vi "Intake Execute.vi"() -> ()   [LabVIEW 2017]
uses:
  Intake Control Type.ctl
  <vilib>/Rock Robotics/WPI/Solenoid/WPI_SolenoidValue.ctl
  <vilib>/Rock Robotics/WPI/DriverStation/WPI_DriverStationRobotMode2.ctl
  Intake Notifier.ctl
  <vilib>/Rock Robotics/WPI/ThirdParty/Phoenix-LabVIEW/Motor Controller/Controls/CTRE_Phoenix_MotorControl_ControlMode.ctl
  Intake Globals.vi
  Utility VIs/Refnum Names.vi
  Robot Global Data.vi
  Lift/Lift Globals.vi
  <vilib>/Rock Robotics/Network Tables/NT Write Boolean.vi
  <vilib>/Rock Robotics/WPI/Solenoid/WPI_SolenoidSetEnum.vi
  Intake Rotation/Intake Rotation Globals.vi
panel:
  in  "Max Out":dbl=0.65 format="%#_13g"
  in  "Arm Out Engaged":bool
  out "error out 3":errorcluster
  out "error out 2":errorcluster
  out "error out":errorcluster
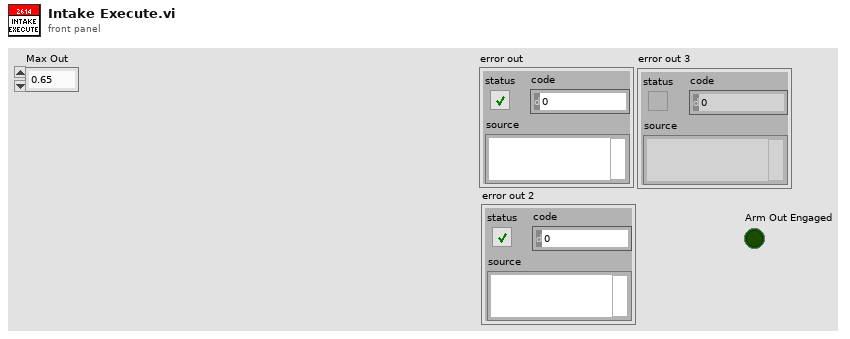
[diagram p1: front panel]
types:
  T1 = typedef "WPI_SolenoidDevRef.ctl" = cluster{"DevStatus":errorcluster, "Pneumatics Control Module":u8, "Forward Solenoid Channel":T2, "Reverse Solenoid Channel":T2}
  T2 = typedef "WPI_SolenoidChannel.ctl" = enum8{"Solenoid 0", "Solenoid 1", "Solenoid 2", "Solenoid 3", "Solenoid 4", "Solenoid 5", "Solenoid 6", "Solenoid 7", "Invalid"}
  T3 = typedef "WPI_MotorControlDeviceRef.ctl" = cluster{"DeviceStatus":errorcluster, "Type":T4, "PWM":cluster{"PWM Channel":T5, "DeadBand":T6}, "CAN":cluster{"Device Number":u8, "SetOutput VI Ref":variant, "GetOutput VI Ref":variant, "Enable VI Ref":variant, "Disable VI Ref":variant, "Data":variant}, "Invert":bool, "DIO PWM":cluster{"PWM \"Enable\" Channel":T5, "DIOChannel":T7, "PWM Rate":dbl}}
  T4 = typedef "WPI_MotorControlType.ctl" = enum16{"PWM", "CAN", "DIO PWM"}
  T5 = typedef "FPGA_DIOPWMChannel.ctl" = enum8{"PWM 0", "PWM 1", "PWM 2", "PWM 3", "PWM 4", "PWM 5", "PWM 6", "PWM 7", "PWM 8", "PWM 9", "PWM MXP 0", "PWM MXP 1", "PWM MXP 2", "PWM MXP 3", "PWM MXP 4", "PWM MXP 5", "PWM MXP 6", "PWM MXP 7", "PWM MXP 8", "PWM MXP 9", "Invalid"}
  T6 = typedef "WPI_PWMDeadband.ctl" = cluster{"Name":string, "maxPositivePwm":i32, "minPositivePwm":i32, "centerPwm":i32, "maxNegativePwm":i32, "minNegativePwm":i32, "angularRange":u16}
  T7 = typedef "FPGA_DIOChannel.ctl" = enum8{"DIO 0", "DIO 1", "DIO 2", "DIO 3", "DIO 4", "DIO 5", "DIO 6", "DIO 7", "DIO 8", "DIO 9", "DIO MXP 0", "DIO MXP 1", "DIO MXP 2", "DIO MXP 3", "DIO MXP 4", "DIO MXP 5", "DIO MXP 6", "DIO MXP 7", "DIO MXP 8", "DIO MXP 9", "DIO MXP 10", "DIO MXP 11", "DIO MXP 12", "DIO MXP 13", "DIO MXP 14", "DIO MXP 15", "SPI Port CS1", "SPI Port CS2", "SPI Port CS3", "SPI Port MISO", "SPI Port MOSI", "Invalid"}
  T8 = typedef "WPI_DriverStationRobotMode2.ctl" = enum16{"Autonomous Disabled", "Autonomous Enabled", "Teleop Disabled", "Teleop Enabled", "Disconnected", "Finish", "Test Disabled", "Test Enabled", "Emergency Stopped"}
  T9 = typedef "WPI_SolenoidValue.ctl" = enum16{"Off", "On", "Forward", "Reverse"}
  T10 = typedef "Intake Control Type.ctl" = enum16{"No Op", "In", "Out", "Test Mode", "Cube_In", "Cube_Out", "State_Change"}
  T11 = typedef "Intake Notifier.ctl" = cluster{"Intake Control Type":T10, "Step":i32, "In":bool, "Speed":dbl, "Out":bool, "Parameter 1":dbl, "Parameter 2":dbl, "Intake Notifier":refnum<notifier>, "Actuate Cube":bool, "Speed In":dbl, "Speed Out":dbl, "Load":bool, "Override":bool, "Exchange":bool, "Intake Open":bool}
  T12 = typedef "CTRE_Phoenix_MotorControl_ControlMode.ctl" = u16
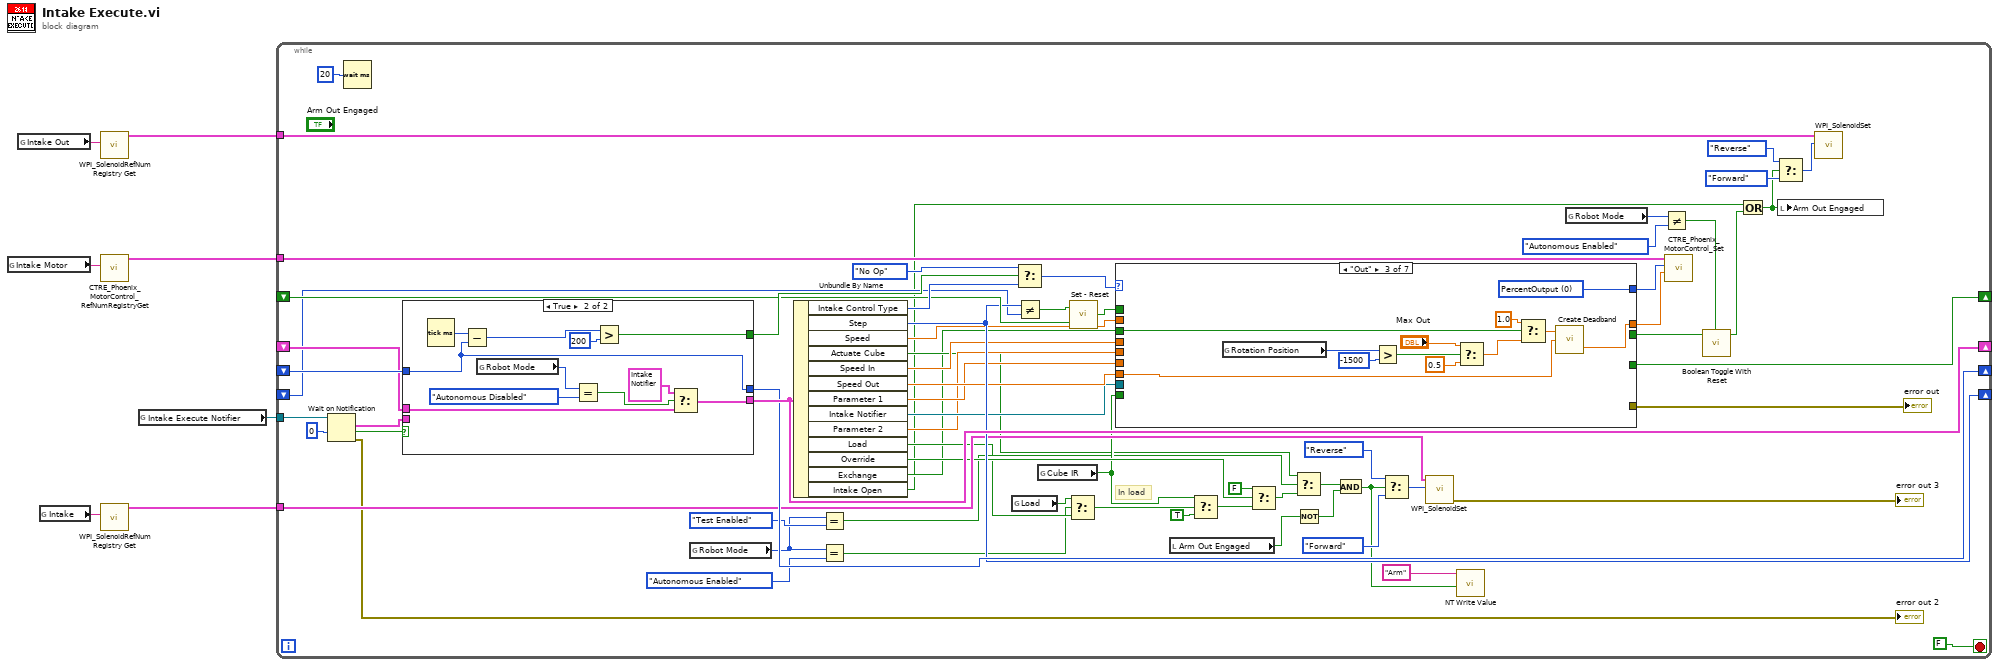
[diagram p0: block diagram]
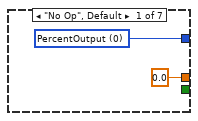
[diagram p2: hidden frame]
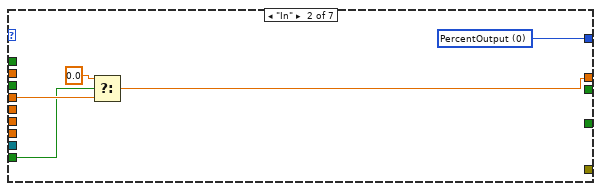
[diagram p3: hidden frame]
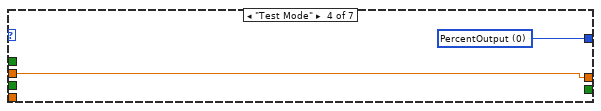
[diagram p4: hidden frame]
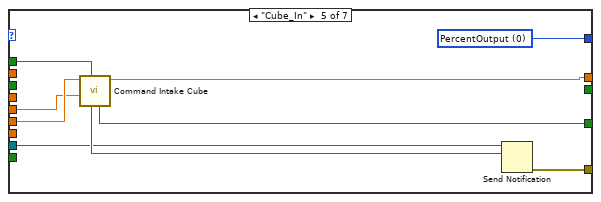
[diagram p5: hidden frame]
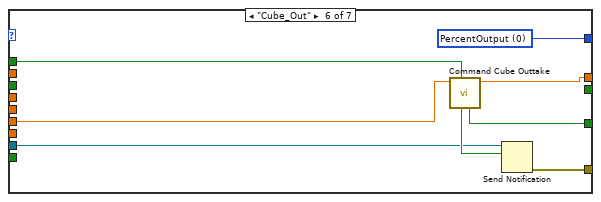
[diagram p6: hidden frame]
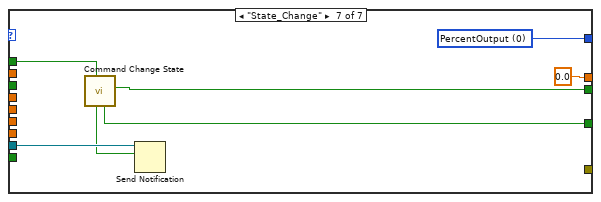
[diagram p7: hidden frame]
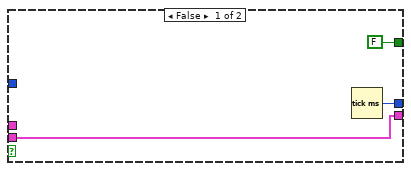
[diagram p8: hidden frame]
diagram:
  n1 = global read "Refnum Names.vi" "Intake Motor"() -> (w6:string)
  n2 = global read "Refnum Names.vi" "Intake Out"() -> (w2:string)
  n3 = global read "Refnum Names.vi" "Intake"() -> (w4:string)
  n4 = call <vilib>:"WPI_SolenoidRefNum Registry Get.vi"("refnum name"=w2) -> ("SolenoidDevRef"=w1:T1)  [unwired: 9 in, 1 out]
  n5 = call <vilib>:"CTRE_Phoenix_MotorControl_RefNumRegistryGet.vi"("refnum name"=w6) -> ("PhoenixMotorControlDevRef"=w5:T3)  [unwired: 9 in, 1 out]
  n6 = call <vilib>:"WPI_SolenoidRefNum Registry Get.vi"("refnum name"=w4) -> ("SolenoidDevRef"=w3:T1)  [unwired: 9 in, 1 out]
  n7 = global read "Intake Globals.vi" "Intake Execute Notifier"() -> (w7:refnum<notifier>)
  n8 = while {
    tunnel: w7 -> [w73]
    shift-right: [w69] -> _
    shift-left: _ -> [w63]
    shift-right: [w67] -> _
    shift-left: _ -> [w68]
    shift-right: [w59] -> _
    shift-left: _ -> [w58]
    shift-right: [w57] -> _
    shift-left: _ -> [w56]
    tunnel: w5 -> [w55]
    tunnel: w3 -> [w51]
    tunnel: w1 -> [w20]
    stop <- FALSE stop-if-true
    # "In load"
    n9 = Wait on Notification(notifier=w73, timeout in ms (-1)=0) -> (notification=w70:T11, timed out?=w71:bool, error out=→"error out 2":errorcluster)  [unwired: 2 in, 1 out]
    n10 = Wait (ms)(milliseconds to wait=u32 20) -> ()  [unwired: 1 out]
    n11 = case shown="True" w71 {
      tunnel: [w122 w129] -> w69
      tunnel: w70 -> [w122 _]
      tunnel: w68 -> [_ w131]
      tunnel: [w123 w131] -> w67
      tunnel: [FALSE w130] -> w64
      tunnel: w63 -> [_ w128]
      frame False {
        n12 = Tick Count (ms)() -> (millisecond timer value=w123:u32)
      }
      frame True {
        n13 = Tick Count (ms)() -> (millisecond timer value=w134:u32)
        n14 = Subtract(x=w134, y=w131) -> (x-y=w133:u32)
        n15 = global read "Robot Global Data.vi" "Robot Mode"() -> (w126:T8)
        n16 = Equal?(x=w126, y=WPI_DriverStationRobotMode2."Autonomous Disabled") -> (x = y?=w124:bool)
        n17 = Greater?(x=w133, y=u32 200) -> (0:w130:bool)
        n18 = Select(t=T11 {"Intake Control Type"=enum."No Op", "Step"=0, "In"=FALSE, "Speed"=0.0, "Out"=FALSE, "Parameter 1"=0.0, "Parameter 2"=0.0, "Intake Notifier"=refnum, "Actuate Cube"=FALSE, "Speed In"=0.0, "Speed Out"=0.0, "Load"=FALSE, "Override"=FALSE, "Exchange"=FALSE, "Intake Open"=FALSE} ("Intake Notifier"), s=w124, f=w128) -> (s? t:f=w129:T11)
      }
    }
    n19 = global read "Robot Global Data.vi" "Robot Mode"() -> (w24:T8)
    n20 = Unbundle By Name(w69) -> ("Intake Control Type"=w65:T10, "Step"=w57:i32, "Speed"=w52:dbl, "Actuate Cube"=w33:bool, "Speed In"=w47:dbl, "Speed Out"=w46:dbl, "Parameter 1"=w45:dbl, "Intake Notifier"=w44:refnum<notifier>, "Parameter 2"=w43:dbl, "Load"=w28:bool, "Override"=w40:bool, "Exchange"=w22:bool, "Intake Open"=w14:bool)
    n21 = Equal?(x=w24, y=WPI_DriverStationRobotMode2."Test Enabled") -> (x = y?=w35:bool)
    n22 = Equal?(x=w24, y=WPI_DriverStationRobotMode2."Autonomous Enabled") -> (x = y?=w25:bool)
    n23 = global read "Lift Globals.vi" "Load"() -> (w23:bool)
    n24 = Select(t=Intake_Control_Type."No Op", s=w64, f=w65) -> (s? t:f=w66:T10)
    n25 = Not Equal?(x=w57, y=w56) -> (x != y?=w61:bool)
    n26 = global read "Intake Globals.vi" "Cube IR"() -> (w39:bool)
    n27 = Select(t=w23, s=w25, f=w28) -> (s? t:f=w27:bool)
    n28 = call "Set - Reset.vi"("Reset"=w58, "Set"=w61) -> ("Output"=w60:bool)
    n29 = case shown="\"Out\"" w66 {
      tunnel: w60 -> [_ _ _ _ w103 w108 w115]
      tunnel: [_ _ _ _ w100 w112 w118] -> w59
      tunnel: [0.0 ("Output") w80 w92 w95 w105 w113 0.0 ("Output")] -> w54
      tunnel: [w76 w82 w94 w96 w104 w107 w120] -> w53
      tunnel: w52 -> [_ _ _ w95 _ _ _]
      tunnel: w47 -> [_ w81 _ _ _ _ _]
      tunnel: w39 -> [_ w79 _ _ _ _ _]
      tunnel: w46 -> [_ _ w93 _ _ _ _]
      tunnel: w45 -> [_ _ _ _ w102 w109 _]
      tunnel: w44 -> [_ _ _ _ w99 w110 w117]
      tunnel: w43 -> [_ _ _ _ w98 _ _]
      tunnel: [_ _ _ _ w97 w106 _] -> w42
      tunnel: w22 -> [_ _ w89 _ _ _ _]
      tunnel: [_ _ _ _ _ _ w114] -> w12
      frame "No Op", Default {
        w76 = T12 0 items=["PercentOutput"=0, "Position"=1, "Velocity"=2, "Current"=3, "Follower"=5, "MotionProfile"=6, "MotionMagic"=7, "MotionMagicArc"=8, "MotionProfileArc"=10, "Disabled"=15] ("Control Mode")
      }
      frame "In" {
        w82 = T12 0 items=["PercentOutput"=0, "Position"=1, "Velocity"=2, "Current"=3, "Follower"=5, "MotionProfile"=6, "MotionMagic"=7, "MotionMagicArc"=8, "MotionProfileArc"=10, "Disabled"=15] ("Control Mode")
        n30 = Select(t=0.0, s=w79, f=w81) -> (s? t:f=w80:dbl)
      }
      frame "Out" {
        w94 = T12 0 items=["PercentOutput"=0, "Position"=1, "Velocity"=2, "Current"=3, "Follower"=5, "MotionProfile"=6, "MotionMagic"=7, "MotionMagicArc"=8, "MotionProfileArc"=10, "Disabled"=15] ("Control Mode")
        n31 = global read "Intake Rotation Globals.vi" "Rotation Position"() -> (w86:i32)
        n32 = Greater?(x=w86, y=-1500) -> (0:w87:bool)
        n33 = Select(t="Max Out", s=w87, f=0.5) -> (s? t:f=w88:dbl)
        n34 = Select(t=1.0, s=w89, f=w88) -> (s? t:f=w91:dbl)
        n35 = call "Create Deadband.vi"("Input"=w93, "Output Upper Limit"=w91) -> ("Output"=w92:dbl)  [unwired: 2 in]
      }
      frame "Test Mode" {
        w96 = T12 0 items=["PercentOutput"=0, "Position"=1, "Velocity"=2, "Current"=3, "Follower"=5, "MotionProfile"=6, "MotionMagic"=7, "MotionMagicArc"=8, "MotionProfileArc"=10, "Disabled"=15] ("Control Mode")
      }
      frame "Cube_In" {
        w104 = T12 0 items=["PercentOutput"=0, "Position"=1, "Velocity"=2, "Current"=3, "Follower"=5, "MotionProfile"=6, "MotionMagic"=7, "MotionMagicArc"=8, "MotionProfileArc"=10, "Disabled"=15] ("Control Mode")
        n36 = call "Command Intake Cube.vi"("Startup"=w103, "Timeout"=w98, "Speed"=w102) -> ("Output"=w105:dbl, "Reinit"=w100:bool, "Completed"=w101:bool)  [unwired: 6 in]
        n37 = Send Notification(notification=w101, notifier=w99) -> (error out=w97:errorcluster)  [unwired: 1 in, 1 out]
      }
      frame "Cube_Out" {
        w107 = T12 0 items=["PercentOutput"=0, "Position"=1, "Velocity"=2, "Current"=3, "Follower"=5, "MotionProfile"=6, "MotionMagic"=7, "MotionMagicArc"=8, "MotionProfileArc"=10, "Disabled"=15] ("Control Mode")
        n38 = call "Command Cube Outtake.vi"("Startup"=w108, "Speed"=w109) -> ("Output"=w113:dbl, "Reinit"=w112:bool, "Completed"=w111:bool)  [unwired: 7 in]
        n39 = Send Notification(notification=w111, notifier=w110) -> (error out=w106:errorcluster)  [unwired: 1 in, 1 out]
      }
      frame "State_Change" {
        w120 = T12 0 items=["PercentOutput"=0, "Position"=1, "Velocity"=2, "Current"=3, "Follower"=5, "MotionProfile"=6, "MotionMagic"=7, "MotionMagicArc"=8, "MotionProfileArc"=10, "Disabled"=15] ("Control Mode")
        n40 = call "Command Change State.vi"("Startup"=w115) -> ("Actuate"=w114:bool, "Reinit"=w118:bool, "Completed"=w116:bool)  [unwired: 8 in]
        n41 = Send Notification(notification=w116, notifier=w117) -> ()  [unwired: 1 in, 2 out]
      }
    }
    "error out" <- w42
    n42 = local read "Arm Out Engaged"() -> (w16:bool)
    n43 = Select(t=w39, s=w27, f=TRUE) -> (s? t:f=w37:bool)
    n44 = Select(t=FALSE, s=w40, f=w37) -> (s? t:f=w34:bool)
    n45 = Select(t=w33, s=w35, f=w34) -> (s? t:f=w32:bool)
    n46 = Not(x=w16) -> (.not. x?=w15:bool)
    n47 = And(x=w32, y=w15) -> (x .and. y?=w17:bool)
    n48 = Select(t=WPI_SolenoidValue."Reverse" ("Value"), s=w17, f=WPI_SolenoidValue."Forward") -> (s? t:f=w50:T9)
    n49 = call-poly <vilib>:"WPI_SolenoidSet.vi"("Value"=w50, "SolenoidDevRef"=w51) -> ("error out"=→"error out 3":errorcluster)  [unwired: 8 in, 1 out]
    n50 = call-poly <vilib>:"NT Write Value.vi"("Boolean"=w17, "Name"="Arm") -> ()  [unwired: 9 in, 1 out]
    n51 = global read "Robot Global Data.vi" "Robot Mode"() -> (w9:T8)
    n52 = Not Equal?(x=w9, y=WPI_DriverStationRobotMode2."Autonomous Enabled") -> (x != y?=w8:bool)
    n53 = call <vilib>:"CTRE_Phoenix_MotorControl_Set.vi"("Output"=w54, "Control Mode"=w53, "PhoenixMotorControlDevRef"=w55) -> ()  [unwired: 7 in, 2 out]
    n54 = call "Boolean Toggle With Reset.vi"("Input"=w12, "Reset"=w8) -> ("Output"=w11:bool)  [unwired: 25 in]
    n55 = Or(x=w14, y=w11) -> (x .or. y?=w13:bool)
    n56 = Select(t=WPI_SolenoidValue."Reverse" ("Value"), s=w13, f=WPI_SolenoidValue."Forward" ("Value")) -> (s? t:f=w21:T9)
    n57 = local write "Arm Out Engaged"(w13) -> ()
    n58 = call-poly <vilib>:"WPI_SolenoidSet.vi"("Value"=w21, "SolenoidDevRef"=w20) -> ()  [unwired: 8 in, 2 out]
  }
